vi "MultiTest.vi"(10 "Array":u8[](array[numeric]), 11 "Data_In":u16 format="%.0b") -> (2 "MaskedWord":u32 format="%016b", 3 "Data_Out":u16 format="%.0b")   [LabVIEW 2017, in "Bit Manipulation.lvlib"]
uses:
  Bit Manipulation.lvlib
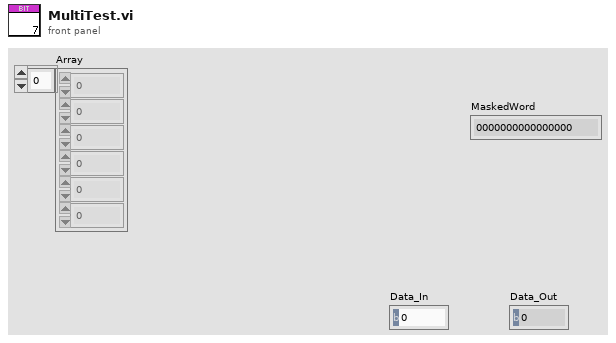
[diagram p1: front panel]
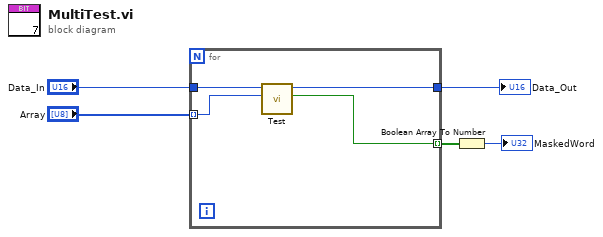
[diagram p0: block diagram]
diagram:
  n1 = for {
    tunnel: "Array" -> [w7] mode=indexing
    tunnel: [w6] -> w3 mode=indexing
    tunnel: "Data_In" -> [w9]
    tunnel: [w8] -> w1
    n2 = call "Test.vi"("Bit to test"=w7, "Data_In"=w9) -> ("bit value"=w6:bool, "Data_Out"=w8:u16)  [unwired: 8 in]
  }
  "Data_Out" <- w1
  n3 = Boolean Array To Number(Boolean array=w3) -> (number=→"MaskedWord":u32)
